vi "Main.vi"() -> ()   [LabVIEW 2024]
uses:
  <vilib>/NI/Modbus Library/API/Master/Modbus Master.lvclass
  Adams Library/6017/Support VIs/Range.ctl
  Adams Library/6224/Support VIs/AO Voltage Range.ctl
  <vilib>/addons/_JKI Toolkits/State Machine/_JKI_lib_State_Machine.llb/Select State(s)_err__jki_lib_state_machine.vi
  <vilib>/numeric/Random Number (Range) DBL.vi
  <vilib>/Utility/file.llb/Write Delimited Spreadsheet (DBL).vi
  <vilib>/Utility/file.llb/Write Delimited Spreadsheet (string).vi
  <userlib>/_OpenG.lib/appcontrol/appcontrol.llb/openg_application_control.lvlib
panel:
  out "Temperature":dbl format="%#_g °C"
  out "ICM Test":dbl(slide)=1.0 scale=0.0..100.0
  in  "Log File Name":string
  in  "Log Data":bool
  in  "Load Enable":bool
  out ">14µ":dbl
  out ">6µ":dbl
  out ">4µ":dbl
  out "Flow Rate":dbl[unit] format="%#_gl/m"
  in  "Load Percentage":u32(slide)=1 scale=0.0..100.0
  out "Post Cooler Temp":dbl format="%#.2g °C"
  out "Load Manifold Temp":dbl format="%#.2g °C"
  out "Motor Temp":dbl format="%#.2g °C"
  out "Load Pressure":dbl format="%#.2g bar"
  out "Cardev Pressure":dbl format="%#.2g bar"
  out "Post Filter Pressure":dbl format="%#.2g bar"
  out "Prefilter Pressure":dbl format="%#.2g bar"
  out "Temperatures":T1(graph) caption="Waveform Chart - Dark"
  in  "Close Button":bool
  out "Pressures":T2(graph) caption="Waveform Chart - Dark"
  # "HPU VALIDATION TEST"
  # "Temperatures"
  # "Pressures"
  # "Load Control"
  # "Flow Meter"
  # "ICM"
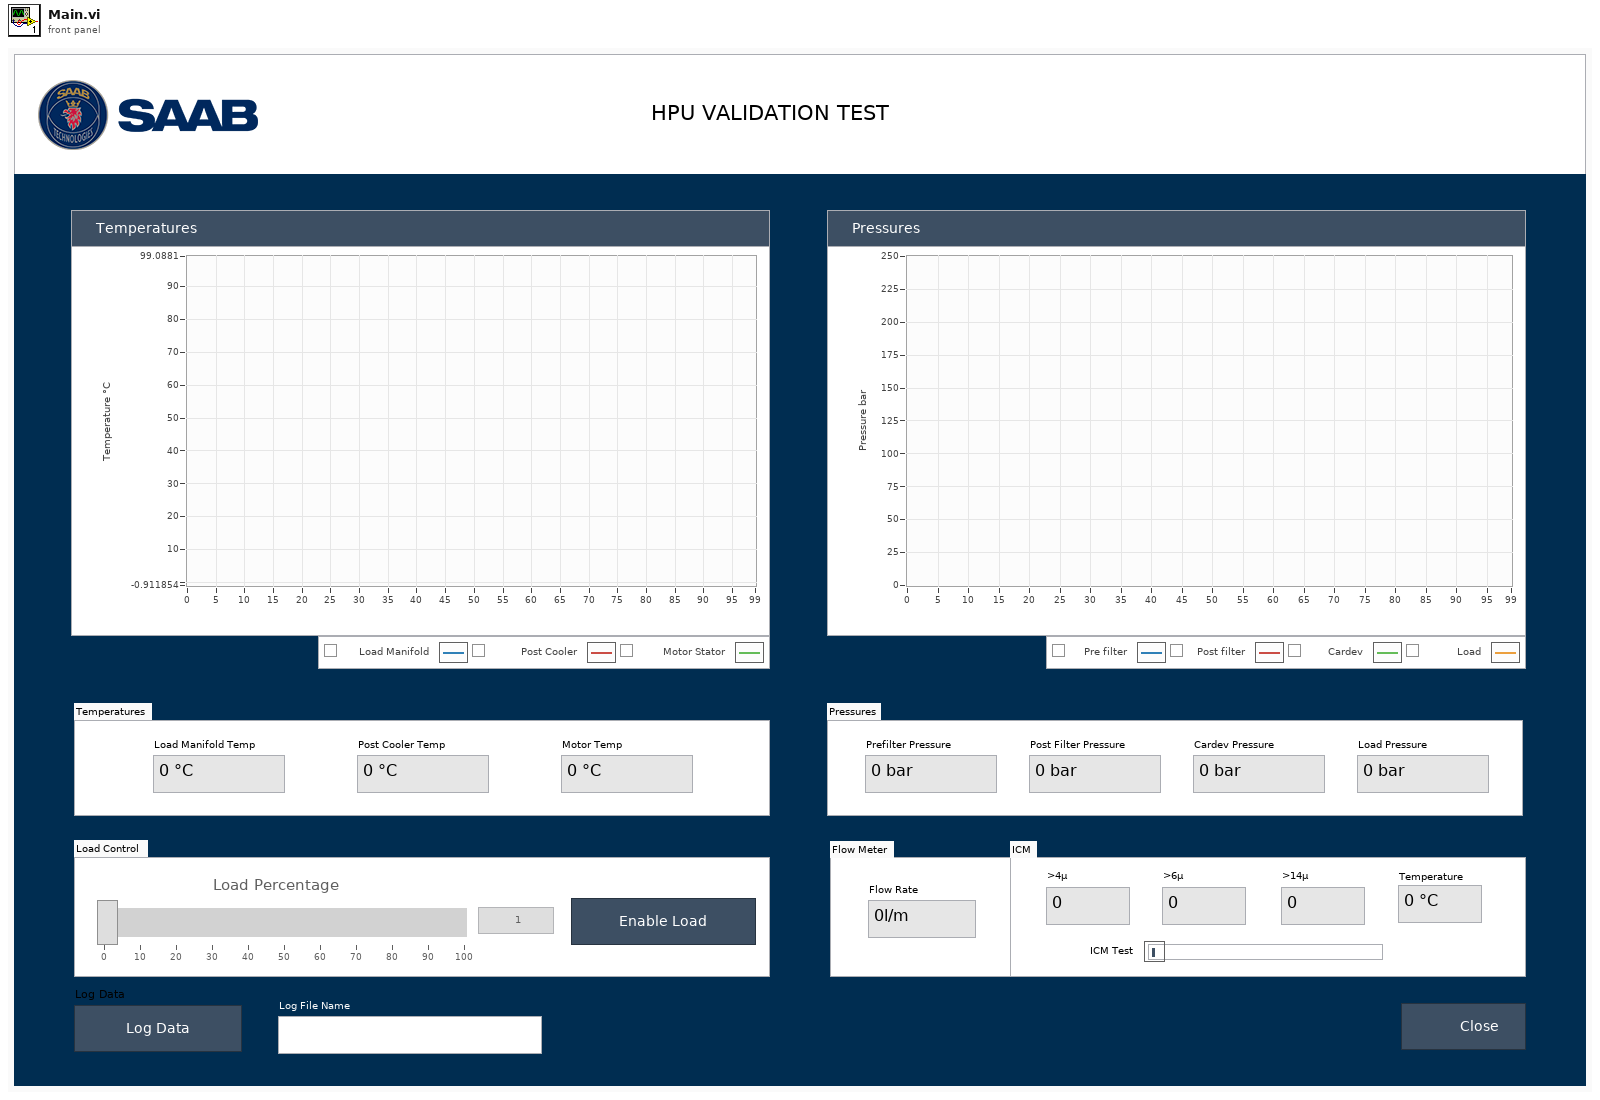
[diagram p1: front panel]
types:
  T1 = cluster{"Numeric":dbl, "Numeric":dbl, "Temperature °C":dbl}
  T2 = cluster{"Pressure bar":dbl, "Pressure bar":dbl, "Pressure bar":dbl, "Pressure bar":dbl}
  T3 = enum32{"Invalid", "Standard", "Closed", "Hidden", "Minimized", "Maximized"}
  T4 = enum32{"invalid app kind", "Development System", "Run Time System", "Student Edition", "Embedded LabVIEW", "Evaluation", "Custom"}
  T5 = cluster{"Numeric":dbl, "Numeric":dbl, "Temperature °C":dbl}[]
  T6 = cluster{"Pressure bar":dbl, "Pressure bar":dbl, "Pressure bar":dbl, "Pressure bar":dbl}[]
  T7 = enum8{"Enabled", "Disabled", "Disabled and Grayed Out"}
  T8 = typedef "Range.ctl" = u16
  T9 = cluster{"Core":cluster{"Current VI Reference":refnum<vi>, "Close Panel on Exit?":bool}, "6017 Ref":refnum<class "Modbus Master.lvclass">, "6224 Ref":refnum<class "Modbus Master.lvclass">, "AI Measurment":dbl[], "Channel Ranges":T8[], "Timestamp":dbl, "Simulate Data":bool, "Results File Path":path, "Log Data":dbl[], "Write Data":bool, "Load Percentage":u32, "ICM Ref":refnum<class "Modbus Master.lvclass">}
  T10 = cluster{"Current VI Reference":refnum<vi>, "Close Panel on Exit?":bool}
  T11 = typedef "AO Voltage Range.ctl" = u16
  T12 = cluster{"Temperature °C":dbl, "Temperature °C":dbl, "Temperature °C":dbl}
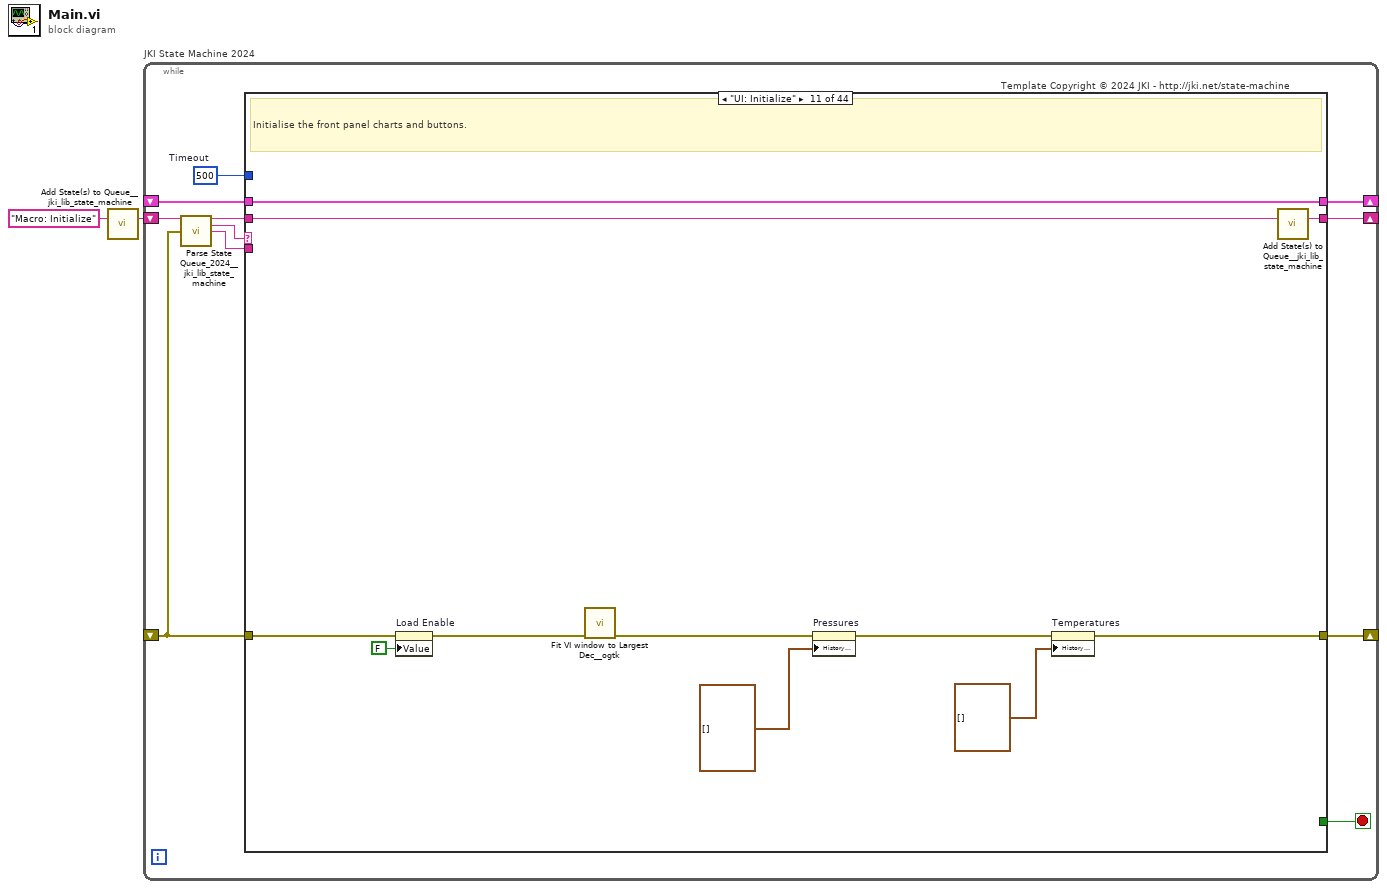
[diagram p0: block diagram]
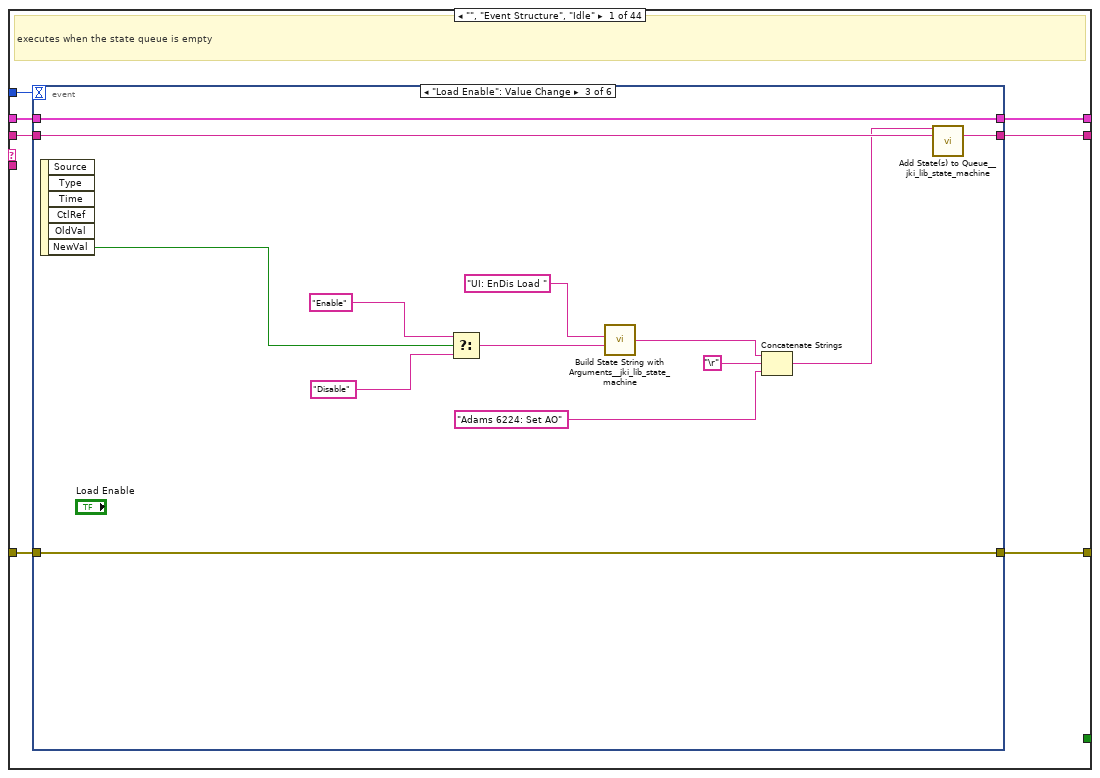
[diagram p2: hidden frame]
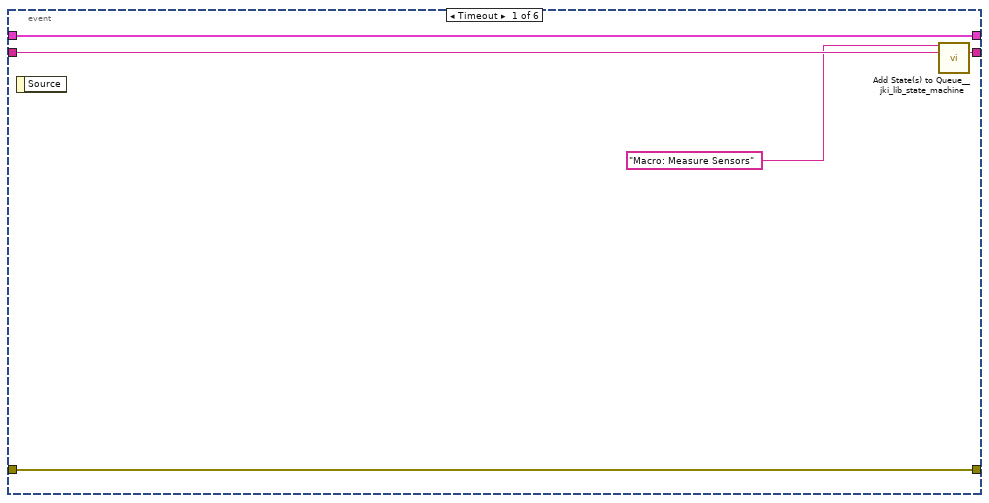
[diagram p3: hidden frame]
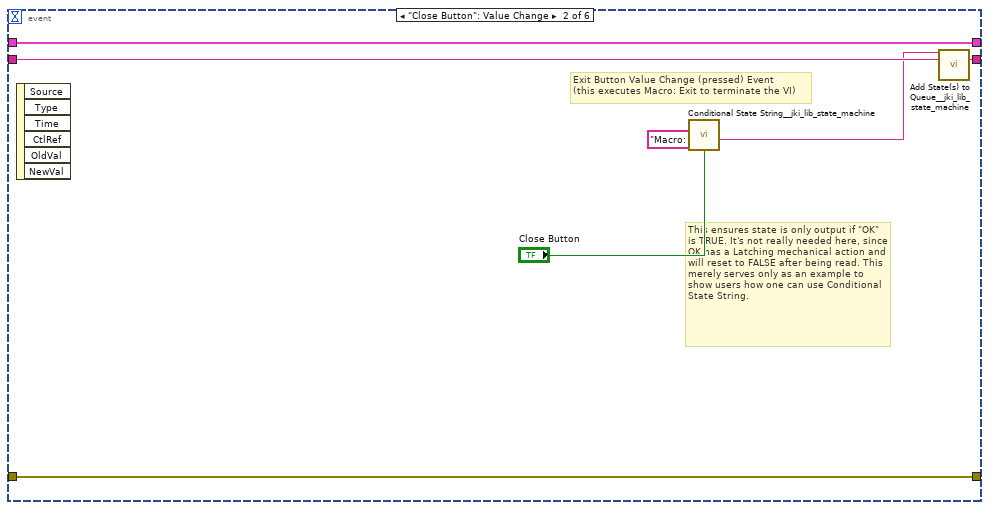
[diagram p4: hidden frame]
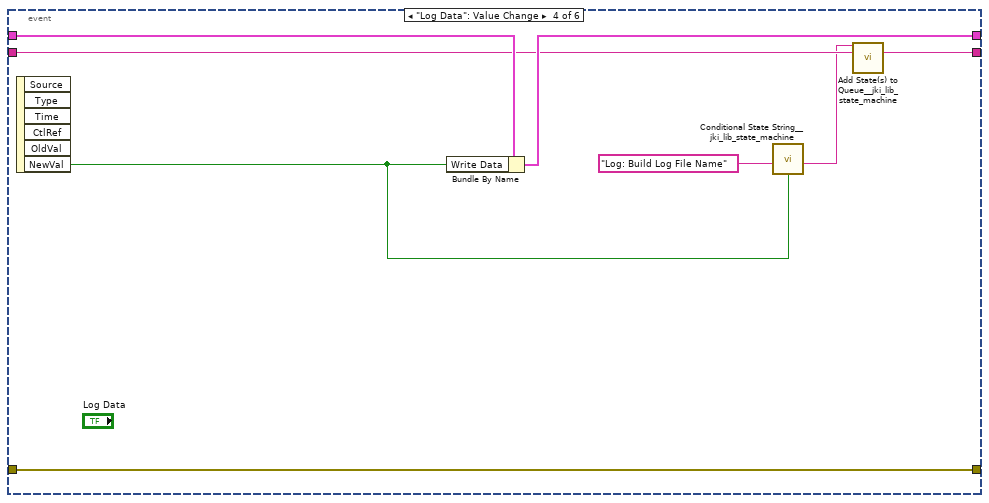
[diagram p5: hidden frame]
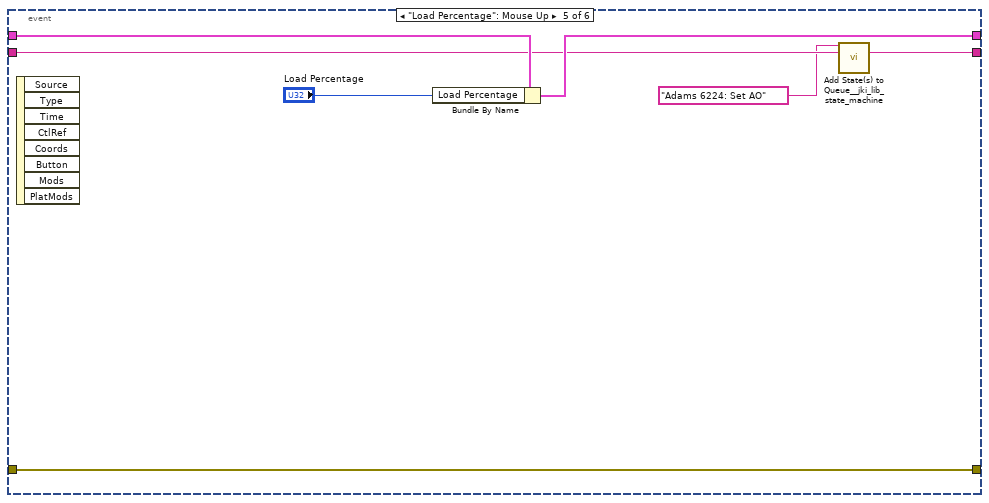
[diagram p6: hidden frame]
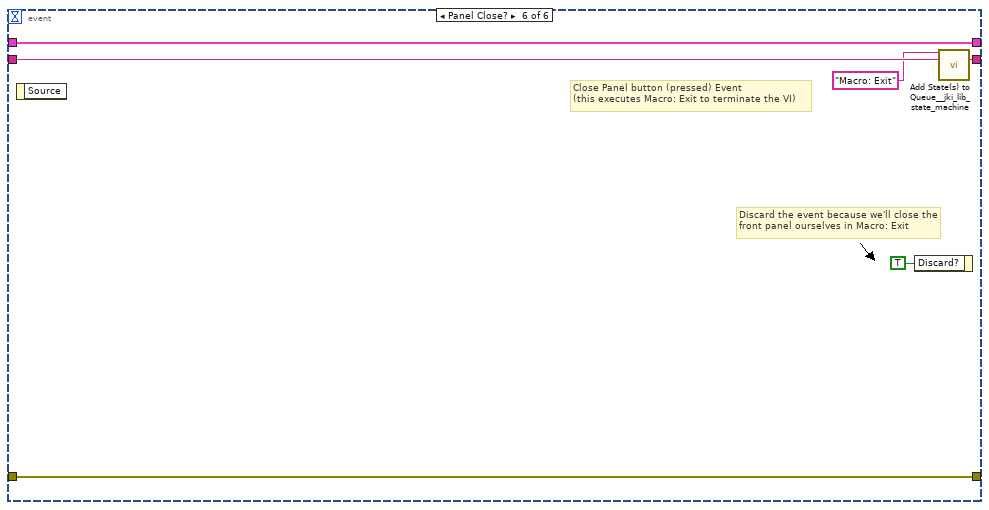
[diagram p7: hidden frame]
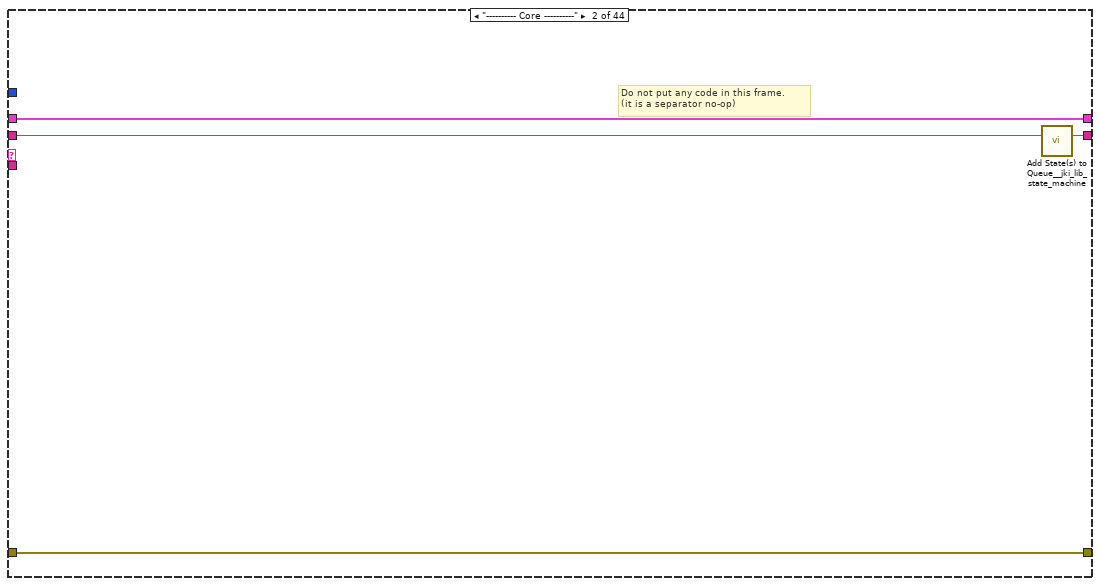
[diagram p8: hidden frame]
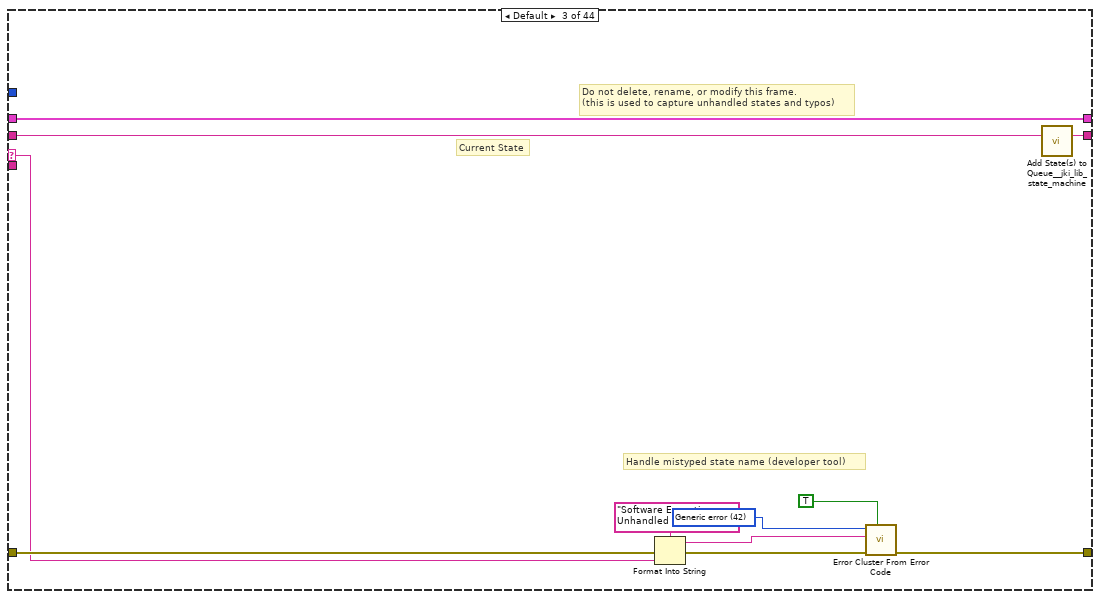
[diagram p9: hidden frame]
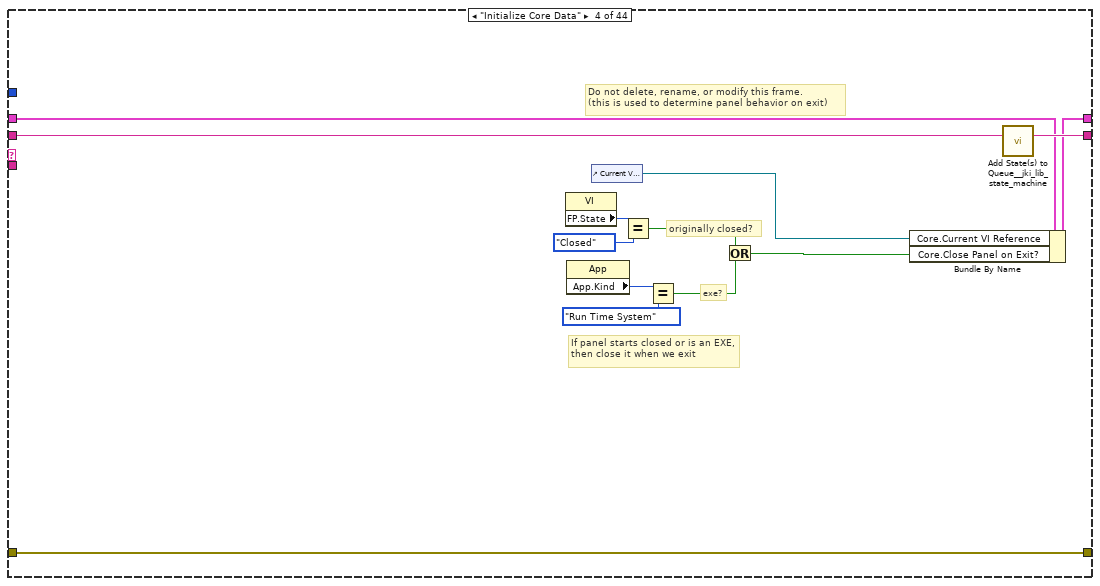
[diagram p10: hidden frame]
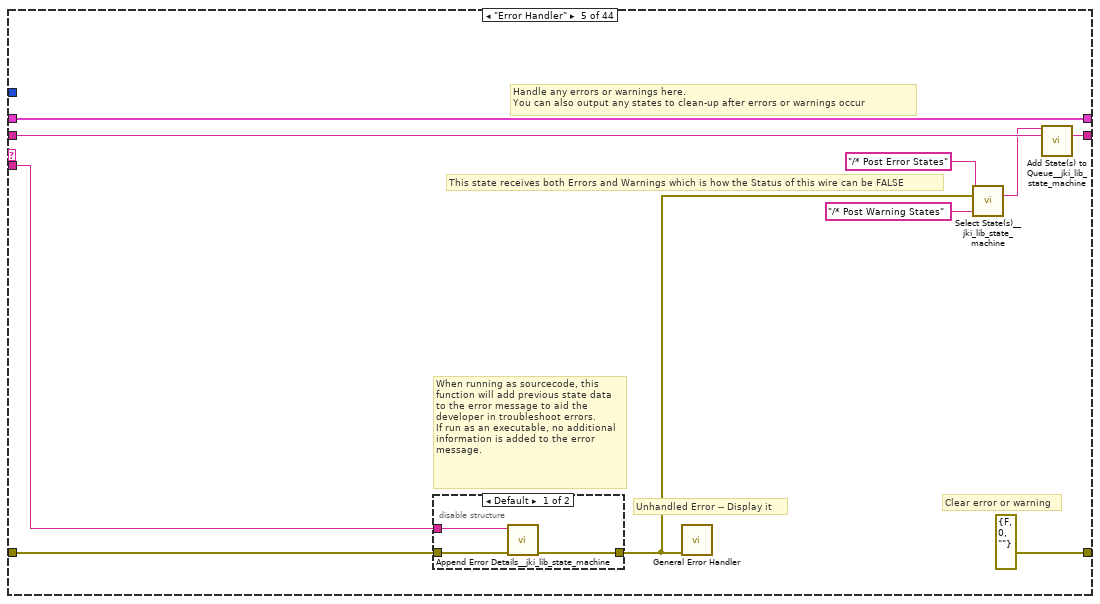
[diagram p11: hidden frame]
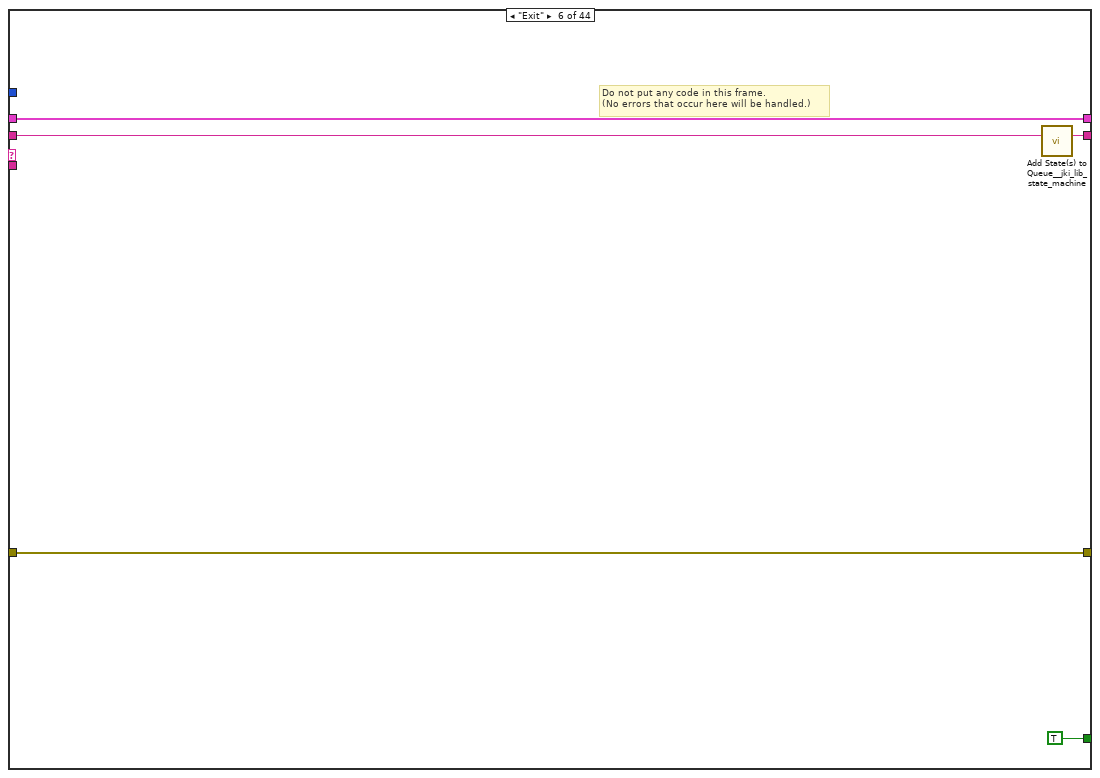
[diagram p13: hidden frame]
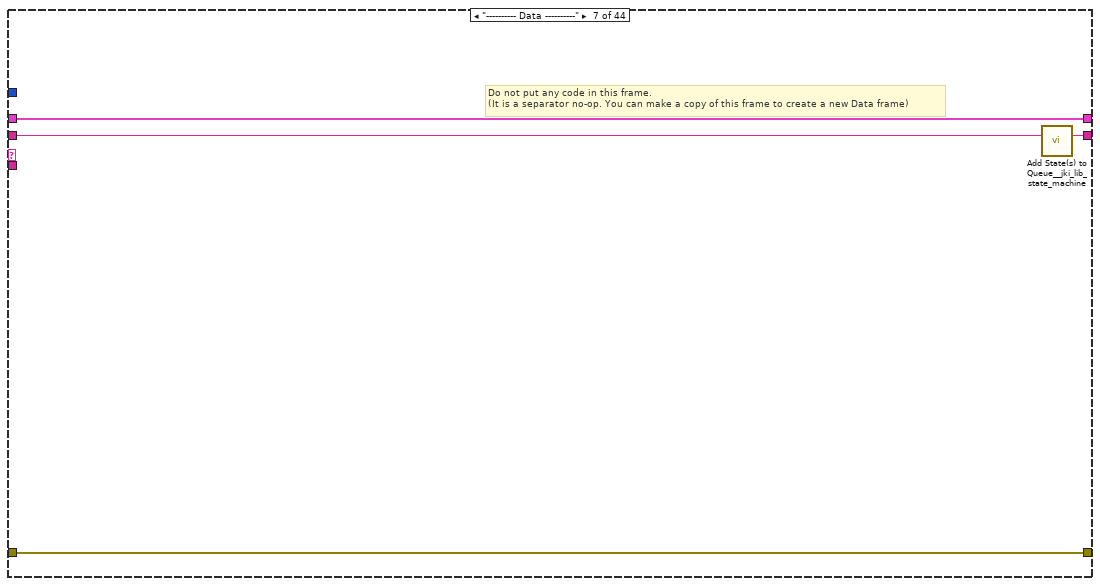
[diagram p14: hidden frame]
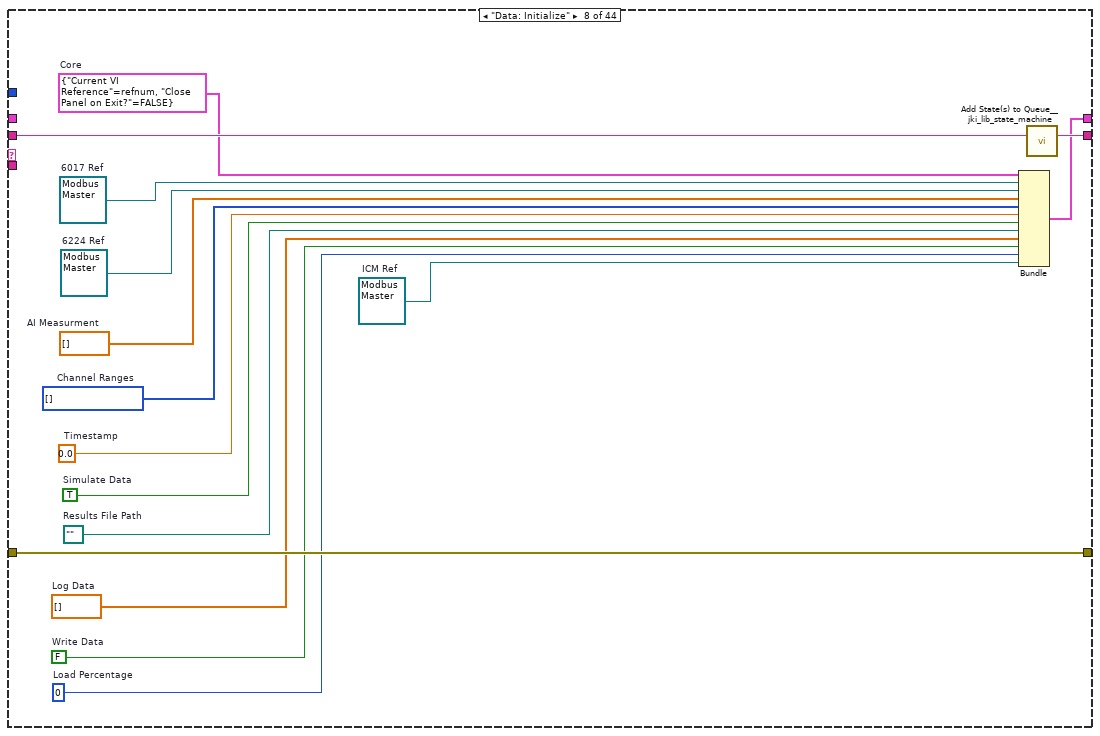
[diagram p15: hidden frame]
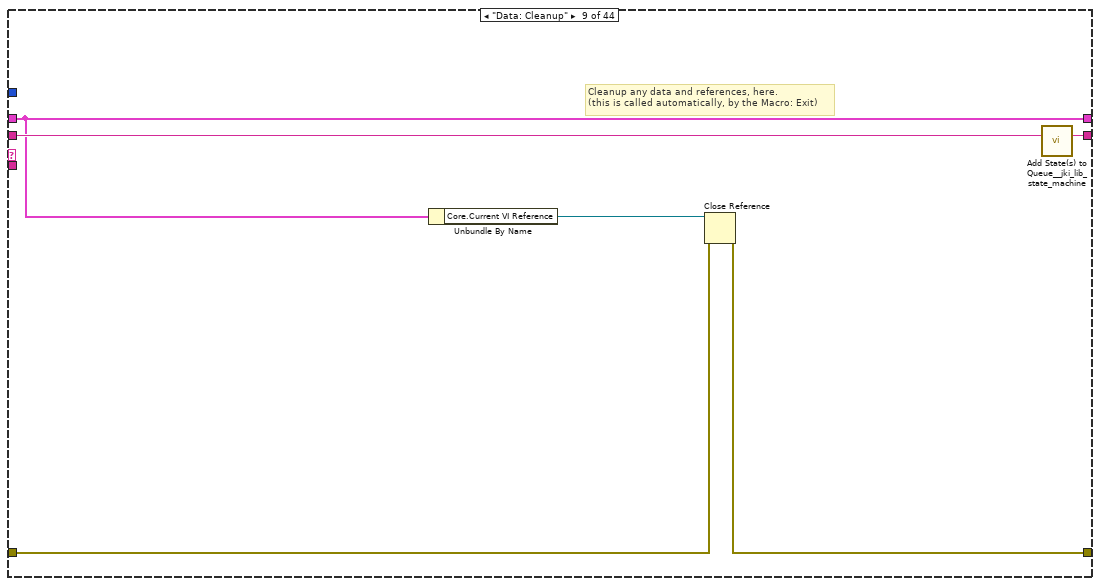
[diagram p16: hidden frame]
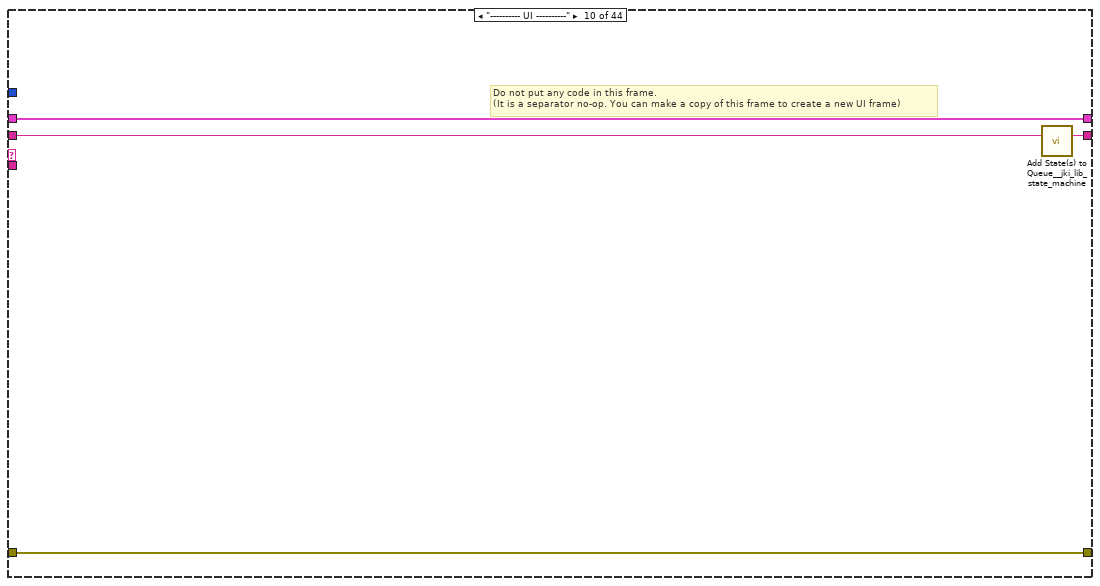
[diagram p17: hidden frame]
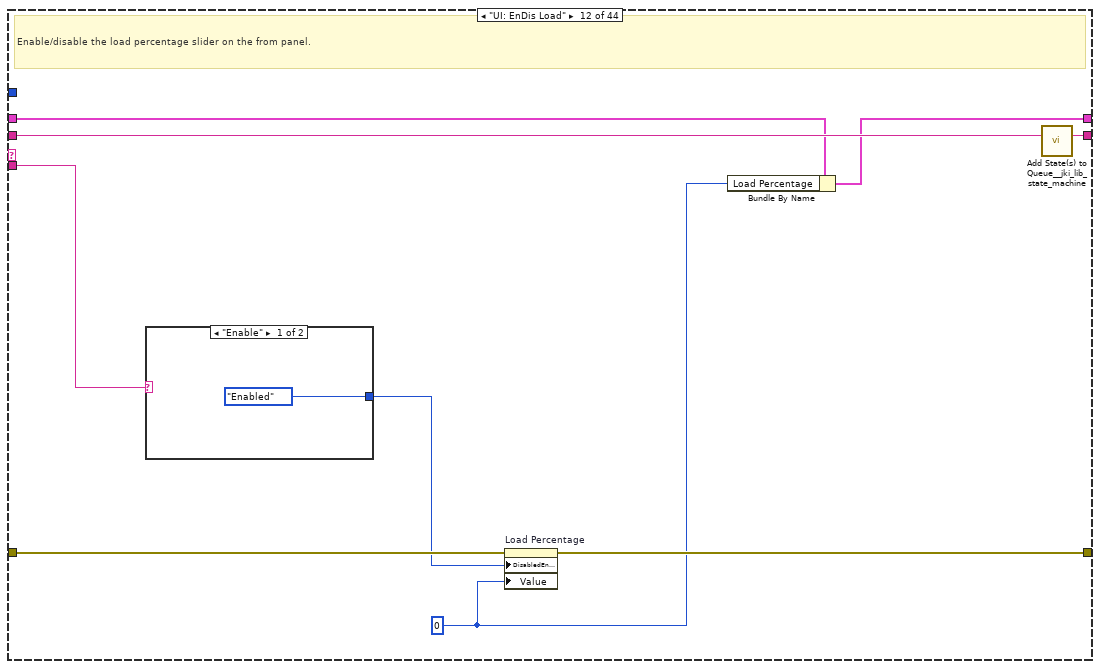
[diagram p18: hidden frame]
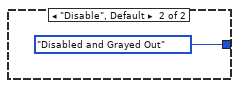
[diagram p19: hidden frame]
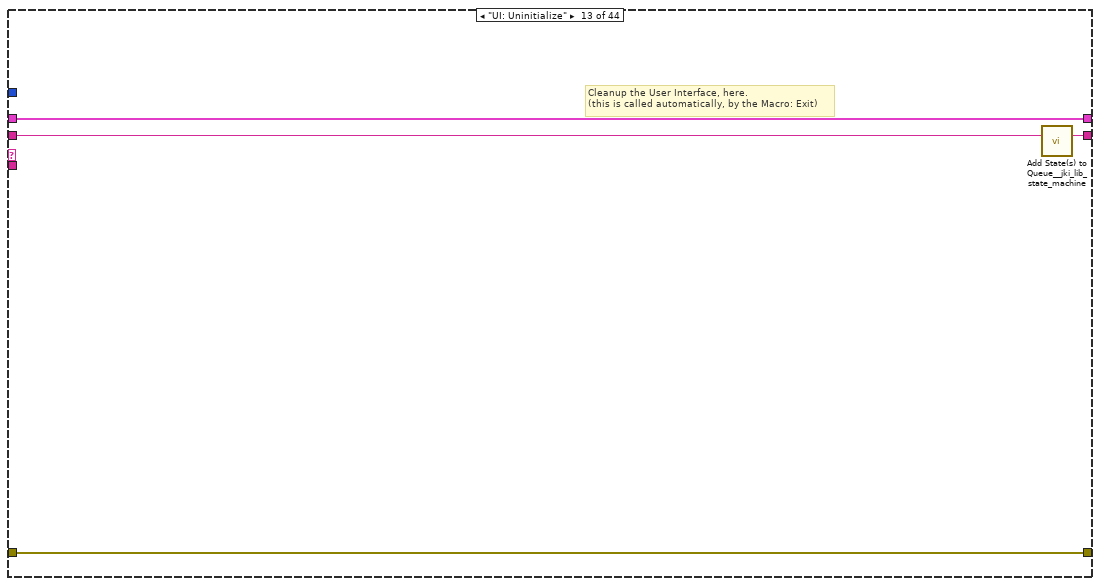
[diagram p20: hidden frame]
diagram:
  n1 = call <vilib>:"Add State(s) to Queue__jki_lib_state_machine.vi"("State(s) in (\"\")"="Macro: Initialize") -> ("States Out"=w2:string)  [unwired: 14 in]
  n2 = while "JKI State Machine 2024" {
    shift-right: [w6] -> _
    shift-left: _ -> [w5]
    shift-right: [w9] -> _
    shift-left: _ -> [w3]
    shift-right: [w8] -> _
    shift-left: w2 -> [w10]
    stop <- w7 stop-if-true
    w4 = 500  # Timeout
    # "Template Copyright © 2024 JKI - http://jki.net/state-machine"
    n3 = call <vilib>:"Parse State Queue_2024__jki_lib_state_machine.vi"("State Queue"=w10, "Error In (no error)"=w3) -> ("Remaining States"=w12:string, "Current State"=w13:string, "Arguments"=w11:string)  [unwired: 11 in]
    n4 = case shown="\"UI: Initialize\"" w13 {
      selector: w13 -> [_ _ w71 _ _ _ _ _ _ _ _ _ _ _ _ _ _ _ _ _ _ _ _ _ _ _ _ _ _ _ _ _ _ _ _ _ _ _ _ _ _ _ _ _]
      tunnel: w12 -> [w20 w70 w75 w94 w104 w113 w117 w133 w139 w143 w154 w163 w169 w175 w186 w255 w260 w265 w274 w278 w286 w299 w373 w384 w396 w400 w408 w424 w432 w436 w455 w459 w476 w480 w488 w496 w509 w518 w527 w531 w541 w564 w568 w572]
      tunnel: w11 -> [_ _ _ _ w99 _ _ _ _ _ _ w158 _ w170 w180 _ _ _ _ _ _ _ _ w376 _ _ _ _ _ _ _ _ _ _ _ _ _ _ _ _ _ _ _ _]
      tunnel: w5 -> [w18 w67 w73 w87 w101 w111 w114 _ w134 w140 w152 w157 w167 w173 w182 w252 w257 w262 w272 w275 w281 w295 w368 w379 w391 w397 w403 w421 w426 w433 w441 w456 w462 w477 w483 w493 w506 w515 w524 w528 w535 w555 w565 w569]
      tunnel: [w17 w68 w77 w91 errorcluster {"status"=FALSE, "code"=0, "source"=""} ("error out") w110 w115 w130 w135 w141 w145 w160 w166 w171 w183 w253 w258 w263 w269 w276 w283 w292 w369 w382 w393 w398 w404 w420 w429 w434 w453 w457 w474 w478 w484 w492 w505 w514 w523 w529 w536 w551 w566 w570] -> w9
      tunnel: w3 -> [w14 w68 w76 w91 w100 w110 w115 w130 w136 w141 w150 w161 w166 w172 w184 w253 w258 w263 w269 w276 w284 w297 w371 w380 w394 w398 w405 w419 w430 w434 w453 w457 w474 w478 w486 w491 w504 w513 w522 w529 w539 w552 w566 w570]
      tunnel: [w19 w69 w74 w93 w103 w112 w116 w132 w138 w142 w153 w162 w168 w174 w185 w254 w259 w264 w273 w277 w285 w298 w372 w383 w395 w399 w407 w423 w431 w435 w454 w458 w475 w479 w487 w495 w508 w517 w526 w530 w540 w563 w567 w571] -> w8
      tunnel: [_ _ _ _ _ TRUE _ _ _ _ _ _ _ _ _ _ _ _ _ _ _ _ _ _ _ _ _ _ _ _ _ _ _ _ _ _ _ _ _ _ _ _ _ _] -> w7
      tunnel: [w16 w67 w73 w92 w101 w111 w114 w131 w134 w140 w152 w156 w167 w173 w182 w252 w257 w262 w272 w275 w280 w294 w367 w377 w390 w397 w402 w422 w425 w433 w440 w456 w461 w477 w482 w494 w507 w516 w525 w528 w534 w554 w565 w569] -> w6
      tunnel: w4 -> [w15 _ _ _ _ _ _ _ _ _ _ _ _ _ _ _ _ _ _ _ _ _ _ _ _ _ _ _ _ _ _ _ _ _ _ _ _ _ _ _ _ _ _ _]
      frame "", "Event Structure", "Idle" {
        # "executes when the state queue is empty"
        n5 = event shown="[2] \"Load Enable\": Value Change" {
          selector: _ -> [_ _ _ _ _ _]
          dyn-events: _ -> [_ _ _ _ _ _]
          timeout: w15 -> [_ _ _ _ _ _]
          tunnel: w20 -> [w25 w32 w43 w49 w55 w66]
          tunnel: [w24 w31 w44 w50 w56 w65] -> w19
          tunnel: w18 -> [w22 w29 w35 w52 w58 w63]
          tunnel: [w23 w30 w45 w53 w60 w64] -> w17
          tunnel: w14 -> [w23 w30 w45 w53 w60 w64]
          tunnel: [w22 w29 w35 w51 w59 w63] -> w16
          event Timeout {
            n6 = event-data() -> ()  [unwired: 1 in, 1 out]
            n7 = call <vilib>:"Add State(s) to Queue__jki_lib_state_machine.vi"("State(s) in Front (\"\")"="Macro: Measure Sensors", "State(s) in (\"\")"=w25) -> ("States Out"=w24:string)  [unwired: 13 in]
          }
          event "Close Button": Value Change {
            # "This ensures state is only output if \"OK\" is TRUE. It's not really needed here, since OK has a Latching mechanical action and will reset to FALSE after being read. This merely serves only as an example to show users how one can use Conditional State String."
            # "Exit Button Value Change (pressed) Event\n(this executes Macro: Exit to terminate the VI)"
            n8 = event-data() -> ()  [unwired: 1 in, 6 out]
            n9 = call <vilib>:"Conditional State String__jki_lib_state_machine.vi"("Do State(s)?"="Close Button", "State"="Macro: Exit") -> ("State Out"=w27:string)  [unwired: 7 in]
            n10 = call <vilib>:"Add State(s) to Queue__jki_lib_state_machine.vi"("State(s) in Front (\"\")"=w27, "State(s) in (\"\")"=w32) -> ("States Out"=w31:string)  [unwired: 13 in]
          }
          event "Load Enable": Value Change {
            n11 = event-data() -> ("NewVal"=w42:bool)  [unwired: 1 in, 5 out]
            n12 = Select(t="Enable", s=w42, f="Disable") -> (s? t:f=w40:string)
            n13 = call <vilib>:"Build State String with Arguments__jki_lib_state_machine.vi"("Arguments (\"\")"=w40, "State"="UI: EnDis Load ") -> ("State with Arguments"=w34:string)  [unwired: 4 in]
            n14 = Concatenate Strings(w34, "\r", "Adams 6224: Set AO") -> (w37:string)
            n15 = call <vilib>:"Add State(s) to Queue__jki_lib_state_machine.vi"("State(s) in Front (\"\")"=w37, "State(s) in (\"\")"=w43) -> ("States Out"=w44:string)  [unwired: 13 in]
          }
          event "Log Data": Value Change {
            n16 = event-data() -> ("NewVal"=w48:bool)  [unwired: 1 in, 5 out]
            n17 = Bundle By Name(cluster=w52, "Write Data"=w48) -> (w51:T9)
            n18 = call <vilib>:"Conditional State String__jki_lib_state_machine.vi"("Do State(s)?"=w48, "State"="Log: Build Log File Name") -> ("State Out"=w46:string)  [unwired: 7 in]
            n19 = call <vilib>:"Add State(s) to Queue__jki_lib_state_machine.vi"("State(s) in Front (\"\")"=w46, "State(s) in (\"\")"=w49) -> ("States Out"=w50:string)  [unwired: 13 in]
          }
          event "Load Percentage": Mouse Up {
            n20 = event-data() -> ()  [unwired: 1 in, 8 out]
            n21 = Bundle By Name(cluster=w58, "Load Percentage"="Load Percentage") -> (w59:T9)
            n22 = call <vilib>:"Add State(s) to Queue__jki_lib_state_machine.vi"("State(s) in Front (\"\")"="Adams 6224: Set AO", "State(s) in (\"\")"=w55) -> ("States Out"=w56:string)  [unwired: 13 in]
          }
          event Panel Close? {
            # "Discard the event because we'll close the front panel ourselves in Macro: Exit"
            # "Close Panel button (pressed) Event\n(this executes Macro: Exit to terminate the VI)"
            n23 = event-data() -> ()  [unwired: 1 in, 1 out]
            n24 = event-data("Discard?"=TRUE) -> ()  [unwired: 1 in, 1 out]
            n25 = call <vilib>:"Add State(s) to Queue__jki_lib_state_machine.vi"("State(s) in Front (\"\")"="Macro: Exit", "State(s) in (\"\")"=w66) -> ("States Out"=w65:string)  [unwired: 13 in]
          }
        }
      }
      frame "---------- Core ----------" {
        # "Do not put any code in this frame.\n(it is a separator no-op)"
        n26 = call <vilib>:"Add State(s) to Queue__jki_lib_state_machine.vi"("State(s) in (\"\")"=w70) -> ("States Out"=w69:string)  [unwired: 14 in]
      }
      frame Default {
        w80 = 42 items=["No error", "Argument error", "Memory is full", "Out of zone", "End of file", "File already open", "Generic file I/O error", "File not found", "File permission error", "Disk is full", "Duplicate path", "Too many files open", "System feature not enabled", "Resource file not found", "Cannot add resource", "Resource not found", "Image not found", "Image memory error", "Pen does not exist", "Config type invalid", "Config token not found", "Config parse error", "Config memory error", "Bad external code format", "Bad external code offset", "External code not present", "Null window", "Destroy window error", "Null menu", "Print aborted", "Bad print record", "Print driver error", "Windows error during printing", "Memory error during printing", "Print dialog error", "Generic print error", "Invalid device refnum", "Device not found", "Device parameter error", "Device unit error", "Cannot open device", "Device call aborted", "Generic error", "Cancelled by user", "Object ID too low", "Object ID too high", "Object not in heap", "Unknown heap", "Unknown object (invalid DefProc)", "Unknown object (DefProc not in table)", "Message out of range", "Invalid (null) method", "Unknown message", "Manager call not supported", "Bad address", "Network operation in progress", "Network operation timed out", "Connection is busy", "Network attribute not supported", "Network error", "Address in use", "System out of memory", "Connection aborted", "Connection refused", "Not connected", "Already connected", "Connection closed", "Initialization error (interapplication manager)", "Bad occurrence", "Wait on unbound occurrence handler", "Occurrence queue overflow", "Datalog type conflict", "Unused", "Unrecognized type (interapplication manager)", "Memory corrupt", "Failed to make temporary DLL", "Old CIN version", "Drag socket not found", "Failed to load drop-object", "Failed to register OLE object", "Failed to release OLE object", "Format specifier type mismatch", "Unknown format specifier", "Too few format specifiers", "Too many format specifiers", "Scan failed", "Newer CIN version", "Error converting to variant", "Runtime menu error", "Password tampered", "Variant attribute not found", "Incompatible variant data type", "Event data is not available", "Event Store is not present", "Occurrence is not found", "Event Queue is not created", "Event info is not available", "Refnum passed is NULL", "Error retrieving Class GUID", "Error retrieving CoClass GUID", "Error retrieving TypeLib GUID.", "Bad built application magic bytes.", "Specific driver is different from the specific driver associated with the Logical Name.", "There is no session opened to the class driver.", "Max Error", "MAX - Error with config objects", "MAX - Error loading configuration", "MAX - Group not supported"]
        # "Current State"
        # "Do not delete, rename, or modify this frame.\n(this is used to capture unhandled states and typos)"
        # "Handle mistyped state name (developer tool)"
        n27 = Format Into String(format string="Software Exception: Unhandled State \"%s\"." ("message"), error in=w76, w71) -> (resulting string=w79:string, error out=w78:errorcluster)  [unwired: 1 in]
        n28 = call <vilib>:"Error Cluster From Error Code.vi"("show call chain? (False)"=TRUE, "error in (no error)"=w78, "error message (\"\")"=w79, "error code (0)"=w80) -> ("error out"=w77:errorcluster)  [unwired: 5 in]
        n29 = call <vilib>:"Add State(s) to Queue__jki_lib_state_machine.vi"("State(s) in (\"\")"=w75) -> ("States Out"=w74:string)  [unwired: 14 in]
      }
      frame "Initialize Core Data" {
        # "Do not delete, rename, or modify this frame.\n(this is used to determine panel behavior on exit)"
        # "originally closed?"
        # "exe?"
        # "If panel starts closed or is an EXE, then close it when we exit"
        n30 = property class="VI"() -> ("FP.State"=w84:T3)  [unwired: 2 in, 2 out]
        n31 = property class="App"() -> ("App.Kind"=w90:T4)  [unwired: 2 in, 2 out]
        n32 = control-ref of="Current VI Reference"() -> (w85:refnum<vi>)
        n33 = Equal?(x=w84, y=T3."Closed" ("Front Panel Window:State")) -> (x = y?=w82:bool)
        n34 = Equal?(x=w90, y=T4."Run Time System" ("Application:Kind")) -> (x = y?=w88:bool)
        n35 = Or(x=w82, y=w88) -> (x .or. y?=w86:bool)
        n36 = Bundle By Name(cluster=w87, "Core.Current VI Reference"=w85, "Core.Close Panel on Exit?"=w86) -> (w92:T9)
        n37 = call <vilib>:"Add State(s) to Queue__jki_lib_state_machine.vi"("State(s) in (\"\")"=w94) -> ("States Out"=w93:string)  [unwired: 14 in]
      }
      frame "Error Handler" {
        # "When running as sourcecode, this function will add previous state data to the error message to aid the developer in troubleshoot errors.\nIf run as an executable, no additional information is added to the error message."
        # "This state receives both Errors and Warnings which is how the Status of this wire can be FALSE"
        # "Unhandled Error -- Display it"
        # "Handle any errors or warnings here.\nYou can also output any states to clean-up after errors or warnings occur"
        # "Clear error or warning"
        n38 = disable-structure shown="Default" {
          disable-tunnel: w100 -> [w107 w108]
          disable-tunnel: w99 -> [w106 _]
          disable-tunnel: [w105 w108] -> w98
          frame condition #0 (active) {
            n39 = call <vilib>:"Append Error Details__jki_lib_state_machine.vi"("error in (no error)"=w107, "Previous State and Argument(s)"=w106) -> ("error out"=w105:errorcluster)  [unwired: 9 in]
          }
          frame condition #1 {
          }
        }
        n40 = call <vilib>:"General Error Handler.vi"("error in (no error)"=w98) -> ()  [unwired: 10 in, 5 out]
        n41 = call-poly <vilib>:"Select State(s)__jki_lib_state_machine.vi"("State(s) if True (\"\")"="/* Post Error States", "Select"=w98, "State(s) if False (\"\")"="/* Post Warning States") -> ("States Out"=w96:string)  [unwired: 12 in]
        n42 = call <vilib>:"Add State(s) to Queue__jki_lib_state_machine.vi"("State(s) in Front (\"\")"=w96, "State(s) in (\"\")"=w104) -> ("States Out"=w103:string)  [unwired: 13 in]
      }
      frame "Exit" {
        # "Do not put any code in this frame.\n(No errors that occur here will be handled.)"
        n43 = call <vilib>:"Add State(s) to Queue__jki_lib_state_machine.vi"("State(s) in (\"\")"=w113) -> ("States Out"=w112:string)  [unwired: 14 in]
      }
      frame "---------- Data ----------" {
        # "Do not put any code in this frame.\n(It is a separator no-op. You can make a copy of this frame to create a new Data frame)"
        n44 = call <vilib>:"Add State(s) to Queue__jki_lib_state_machine.vi"("State(s) in (\"\")"=w117) -> ("States Out"=w116:string)  [unwired: 14 in]
      }
      frame "Data: Initialize" {
        w118 = refnum<class "Modbus Master.lvclass"> refnum  # ICM Ref
        w119 = u32 0  # Load Percentage
        w120 = FALSE  # Write Data
        w121 = dbl[] []  # Log Data
        w122 = path ""  # Results File Path
        w123 = TRUE  # Simulate Data
        w124 = 0.0  # Timestamp
        w125 = T8[] [] items=["+-150mV"=259, "+-500mV"=260, "0~150mV"=261, "0~500mV"=262, "+-1V"=320, "+-5V"=322, "+-10V"=323, "0~1V"=325, "0~5V"=327, "0~10V"=328, "+-20mA"=385, "4~20mA"=384, "0~20mA"=386]  # Channel Ranges
        w126 = dbl[] []  # AI Measurment
        w127 = refnum<class "Modbus Master.lvclass"> refnum  # 6224 Ref
        w128 = refnum<class "Modbus Master.lvclass"> refnum  # 6017 Ref
        w129 = T10 {"Current VI Reference"=refnum, "Close Panel on Exit?"=FALSE}  # Core
        n45 = Bundle("Core"=w129, "6017 Ref"=w128, "6224 Ref"=w127, "AI Measurment"=w126, "Channel Ranges"=w125, "Timestamp"=w124, "Simulate Data"=w123, "Results File Path"=w122, "Log Data"=w121, "Write Data"=w120, "Load Percentage"=w119, "ICM Ref"=w118) -> (w131:T9)  [unwired: 1 in]
        n46 = call <vilib>:"Add State(s) to Queue__jki_lib_state_machine.vi"("State(s) in (\"\")"=w133) -> ("States Out"=w132:string)  [unwired: 14 in]
      }
      frame "Data: Cleanup" {
        # "Cleanup any data and references, here.\n(this is called automatically, by the Macro: Exit)"
        n47 = Unbundle By Name(w134) -> ("Core.Current VI Reference"=w137:refnum<vi>)
        n48 = Close Reference(reference=w137, error in (no error)=w136) -> (error out=w135:errorcluster)
        n49 = call <vilib>:"Add State(s) to Queue__jki_lib_state_machine.vi"("State(s) in (\"\")"=w139) -> ("States Out"=w138:string)  [unwired: 14 in]
      }
      frame "---------- UI ----------" {
        # "Do not put any code in this frame.\n(It is a separator no-op. You can make a copy of this frame to create a new UI frame)"
        n50 = call <vilib>:"Add State(s) to Queue__jki_lib_state_machine.vi"("State(s) in (\"\")"=w143) -> ("States Out"=w142:string)  [unwired: 14 in]
      }
      frame "UI: Initialize" {
        # "Initialise the front panel charts and buttons."
        n51 = property on="Load Enable" class="Bool (strict)"(error in=w150, "Value"=FALSE ("Load Enable")) -> (error out=w151:errorcluster)  [unwired: 1 in, 1 out]
        n52 = call <userlib>:"Fit VI window to Largest Dec__ogtk.vi"("error in (no error)"=w151) -> ("error out"=w148:errorcluster)  [unwired: 5 in, 1 out]
        n53 = property on="Pressures" class="WFChart (strict)"(error in=w148, "History Data"=T6 []) -> (error out=w146:errorcluster)  [unwired: 1 in, 1 out]
        n54 = property on="Temperatures" class="WFChart (strict)"(error in=w146, "History Data"=T5 []) -> (error out=w145:errorcluster)  [unwired: 1 in, 1 out]
        n55 = call <vilib>:"Add State(s) to Queue__jki_lib_state_machine.vi"("State(s) in (\"\")"=w154) -> ("States Out"=w153:string)  [unwired: 14 in]
      }
      frame "UI: EnDis Load" {
        w155 = u32 0 ("Load Percentage")
        # "Enable/disable the load percentage slider on the from panel."
        n56 = case shown="\"Enable\"" w158 {
          tunnel: [T7."Enabled" ("Disabled") T7."Disabled and Grayed Out" ("Disabled")] -> w159
          frame "Enable" {
          }
          frame "Disable", Default {
          }
        }
        n57 = property on="Load Percentage" class="Slide (strict)"(error in=w161, "DisabledEnum"=w159, "Value"=w155) -> (error out=w160:errorcluster)  [unwired: 1 in, 1 out]
        n58 = Bundle By Name(cluster=w157, "Load Percentage"=w155) -> (w156:T9)
        n59 = call <vilib>:"Add State(s) to Queue__jki_lib_state_machine.vi"("State(s) in (\"\")"=w163) -> ("States Out"=w162:string)  [unwired: 14 in]
      }
      frame "UI: Uninitialize" {
        # "Cleanup the User Interface, here.\n(this is called automatically, by the Macro: Exit)"
        n60 = call <vilib>:"Add State(s) to Queue__jki_lib_state_machine.vi"("State(s) in (\"\")"=w169) -> ("States Out"=w168:string)  [unwired: 14 in]
      }
      frame "UI: Cursor Set" {
        # "Argument"
        # "Set and Unset Cursor Busy.\n(Usage: \"UI: Cursor Set >> Busy|Idle\")"
        n61 = case shown="\"Idle\", Default" w170 {
          tunnel: w172 -> [w177 w179]
          tunnel: [w176 w178] -> w171
          frame "Idle", Default {
            n62 = call <vilib>:"Unset Busy.vi"("error in (no error)"=w177) -> ("error out"=w176:errorcluster)  [unwired: 10 in]
          }
          frame "Busy" {
            n63 = call <vilib>:"Set Busy.vi"("error in (no error)"=w179) -> ("error out"=w178:errorcluster)  [unwired: 9 in, 1 out]
          }
        }
        n64 = call <vilib>:"Add State(s) to Queue__jki_lib_state_machine.vi"("State(s) in (\"\")"=w175) -> ("States Out"=w174:string)  [unwired: 14 in]
      }
      frame "UI: Front Panel State" {
        # "Argument"
        # "Set Front Panel Open or Closed\n(Usage: \"UI: Front Panel State >> Open|Close\")"
        n65 = Unbundle By Name(w182) -> ("Core.Current VI Reference"=w181:refnum<vi>)
        n66 = case shown="\"Minimize\", \"Minimized\"" w180 {
          tunnel: w184 -> [w192 w207 w218 w231 w244]
          tunnel: [w194 w208 w220 w233 w246] -> w183
          tunnel: w181 -> [w193 w205 w219 w232 w245]
          frame "Open", "Standard", Default {
            w187 = T3."Standard" ("State")
            n67 = property class="VI"(reference=w193, error in=w192) -> (reference out=w190:refnum<vi>, error out=w191:errorcluster, "FP.State"=w189:T3)
            n68 = Not Equal?(x=w189, y=w187) -> (x != y?=w188:bool)
            n69 = case shown="True" w188 {
              tunnel: [w198 w200] -> w194
              tunnel: w191 -> [w197 w200]
              tunnel: w190 -> [w196 _]
              tunnel: w187 -> [w195 _]
              frame True {
                n70 = invoke class="VI" method="FP.Open"(reference=w196, error in=w197, "Activate"=TRUE, "State"=w195) -> (error out=w198:errorcluster)  [unwired: 1 in, 4 out]
              }
              frame False {
              }
            }
          }
          frame "Close", "Closed" {
            n71 = property class="VI"(reference=w205, error in=w207) -> (reference out=w204:refnum<vi>, error out=w206:errorcluster, "FP.State"=w202:T3)
            n72 = Not Equal?(x=w202, y=T3."Closed" ("Front Panel Window:State")) -> (x != y?=w201:bool)
            n73 = case shown="True" w201 {
              tunnel: [w209 w212] -> w208
              tunnel: w206 -> [w209 w211]
              tunnel: w204 -> [_ w210]
              frame False {
              }
              frame True {
                n74 = invoke class="VI" method="FP.Close"(reference=w210, error in=w211) -> (error out=w212:errorcluster)  [unwired: 1 in, 2 out]
              }
            }
          }
          frame "Hidden", "Hide" {
            w213 = T3."Hidden" ("State")
            n75 = property class="VI"(reference=w219, error in=w218) -> (reference out=w216:refnum<vi>, error out=w217:errorcluster, "FP.State"=w215:T3)
            n76 = Not Equal?(x=w215, y=w213) -> (x != y?=w214:bool)
            n77 = case shown="True" w214 {
              tunnel: [w224 w225] -> w220
              tunnel: w217 -> [w223 w225]
              tunnel: w216 -> [w222 _]
              tunnel: w213 -> [w221 _]
              frame True {
                n78 = invoke class="VI" method="FP.Open"(reference=w222, error in=w223, "State"=w221) -> (error out=w224:errorcluster)  [unwired: 2 in, 4 out]
              }
              frame False {
              }
            }
          }
          frame "Minimize", "Minimized" {
            w226 = T3."Minimized" ("State")
            n79 = property class="VI"(reference=w232, error in=w231) -> (reference out=w229:refnum<vi>, error out=w230:errorcluster, "FP.State"=w228:T3)
            n80 = Not Equal?(x=w228, y=w226) -> (x != y?=w227:bool)
            n81 = case shown="True" w227 {
              tunnel: [w237 w238] -> w233
              tunnel: w230 -> [w236 w238]
              tunnel: w229 -> [w235 _]
              tunnel: w226 -> [w234 _]
              frame True {
                n82 = invoke class="VI" method="FP.Open"(reference=w235, error in=w236, "State"=w234) -> (error out=w237:errorcluster)  [unwired: 2 in, 4 out]
              }
              frame False {
              }
            }
          }
          frame "Maximize", "Maximized" {
            w239 = T3."Maximized" ("State")
            n83 = property class="VI"(reference=w245, error in=w244) -> (reference out=w242:refnum<vi>, error out=w243:errorcluster, "FP.State"=w241:T3)
            n84 = Not Equal?(x=w241, y=w239) -> (x != y?=w240:bool)
            n85 = case shown="True" w240 {
              tunnel: [w250 w251] -> w246
              tunnel: w243 -> [w249 w251]
              tunnel: w242 -> [w248 _]
              tunnel: w239 -> [w247 _]
              frame True {
                n86 = invoke class="VI" method="FP.Open"(reference=w248, error in=w249, "State"=w247) -> (error out=w250:errorcluster)  [unwired: 2 in, 4 out]
              }
              frame False {
              }
            }
          }
        }
        n87 = call <vilib>:"Add State(s) to Queue__jki_lib_state_machine.vi"("State(s) in (\"\")"=w186) -> ("States Out"=w185:string)  [unwired: 14 in]
      }
      frame "---------- Macro ----------" {
        # "Do not put any code in this frame.\n(It is a separator no-op. You can make a copy of this frame to create a new Macro frame)"
        n88 = call <vilib>:"Add State(s) to Queue__jki_lib_state_machine.vi"("State(s) in (\"\")"=w255) -> ("States Out"=w254:string)  [unwired: 14 in]
      }
      frame "Macro: Initialize" {
        w256 = "Data: Initialize\nInitialize Core Data\nUI: Initialize\nUI: EnDis Load>>Disable\nUI: Front Panel State >> Open\nAdams 6224: Init"  # Data: Initialize Initialize Core Data UI: Initialize UI: EnDis Load>>Disable UI: Front Panel State >> Open Adams 6224: Init
        # "Initialization Macro\n(This is called once, when the VI starts)"
        n89 = call <vilib>:"Add State(s) to Queue__jki_lib_state_machine.vi"("State(s) in Front (\"\")"=w256, "State(s) in (\"\")"=w260) -> ("States Out"=w259:string)  [unwired: 13 in]
      }
      frame "Macro: Measure Sensors" {
        # "Sequence for measuring sensors, converting to correct values and logging results (if required)."
        n90 = call <vilib>:"Add State(s) to Queue__jki_lib_state_machine.vi"("State(s) in Front (\"\")"="Adams 6017: Read AI\nPressure: Calculate Pressures\nTemperature: Calculate Temps\nLog: Write Data", "State(s) in (\"\")"=w265) -> ("States Out"=w264:string)  [unwired: 13 in]
      }
      frame "Macro: Exit" {
        # "Exit Macro\n(This is called once, when the VI exits)"
        n91 = Unbundle By Name(w272) -> ("Core.Close Panel on Exit?"=w267:bool)
        n92 = call <vilib>:"Conditional State String__jki_lib_state_machine.vi"("Do State(s)?"=w267, "State"="UI: Front Panel State >> Close") -> ("State Out"=w266:string)  [unwired: 7 in]
        n93 = call <vilib>:"Add State(s) to Queue__jki_lib_state_machine.vi"("State(s) in (\"\")"=w266, "State(s) at Back (\"\")"="Adams 6224: Close\nUI: Uninitialize\nData: Cleanup\nExit") -> ("States Out"=w270:string)  [unwired: 13 in]
        n94 = call <vilib>:"Add State(s) to Queue__jki_lib_state_machine.vi"("State(s) in Front (\"\")"=w270, "State(s) in (\"\")"=w274) -> ("States Out"=w273:string)  [unwired: 13 in]
      }
      frame "---------- Adams 6017 ----------" {
        # "Template Separator\n(You can make a copy of, or modify, this frame)"
        n95 = call <vilib>:"Add State(s) to Queue__jki_lib_state_machine.vi"("State(s) in (\"\")"=w278) -> ("States Out"=w277:string)  [unwired: 14 in]
      }
      frame "Adams 6017: Init" {
        # "#6017 IP address"
        # "Initialise the modbus connection to the Adams 6017 module"
        n96 = call "Adams Connect.vi"("Module Address"="IP address of 6017", "error in (no error)"=w284) -> ("Module Ref"=w279:refnum<class "Modbus Master.lvclass">, "error out"=w283:errorcluster)  [unwired: 12 in]
        n97 = Bundle By Name(cluster=w281, "6017 Ref"=w279) -> (w280:T9)
        n98 = call <vilib>:"Add State(s) to Queue__jki_lib_state_machine.vi"("State(s) in (\"\")"=w286) -> ("States Out"=w285:string)  [unwired: 14 in]
      }
      frame "Adams 6017: Read AI" {
        # "Read back AI register and convert to correct voltage/current values. Record a timestamp for logging purposes."
        n99 = Unbundle By Name(w295) -> ("Channel Ranges"=w288:T8[], "6017 Ref"=w296:refnum<class "Modbus Master.lvclass">, "Simulate Data"=w287:bool)
        n100 = case shown="False" w287 {
          tunnel: w297 -> [w307 w357]
          tunnel: w296 -> [w306 w358]
          tunnel: [w305 w358] -> w293
          tunnel: w288 -> [w303 _]
          tunnel: [w301 w356] -> w292
          tunnel: [w300 w354] -> w291
          frame False {
            n101 = call "Get AI.vi"("Module Ref"=w306, "error in (no error)"=w307) -> ("Modbus master out"=w305:refnum<class "Modbus Master.lvclass">, "AI Measurment"=w302:u16[], "error out"=w304:errorcluster)  [unwired: 11 in]
            n102 = for {
              tunnel: w304 -> [w310]
              tunnel: w303 -> [w312] mode=indexing
              tunnel: w302 -> [w311] mode=indexing
              tunnel: [w309] -> w301
              tunnel: [w308] -> w300 mode=indexing
              # "Use the range register value to convert the \nAI register value to the correct voltage/current"
              n103 = case shown="386" w312 {
                tunnel: w311 -> [_ w317 w320 w323 w326 w329 w332 w335 w338 w341 w344 w347 w350 w352]
                tunnel: w310 -> [w314 w315 w318 w321 w324 w327 w330 w333 w336 w339 w342 w345 w348 w353]
                tunnel: [w314 w315 w318 w321 w324 w327 w330 w333 w336 w339 w342 w345 w348 w353] -> w309
                tunnel: [0.0 ("Current mA") w316 w319 w322 w325 w328 w331 w334 w337 w340 w343 w346 w349 w351] -> w308
                frame 0, Default {
                }
                frame 259 {
                  n104 = call "+-150mV Conv.vi"("Register Value"=w317) -> ("Voltage mV"=w316:dbl)
                }
                frame 260 {
                  n105 = call "+-500mV Conv.vi"("Register Value"=w320) -> ("Voltage mV"=w319:dbl)
                }
                frame 261 {
                  n106 = call "0~150mV Conv.vi"("Register Value"=w323) -> ("Voltage mV"=w322:dbl)
                }
                frame 262 {
                  n107 = call "0~500mV Conv.vi"("Register Value"=w326) -> ("Voltage mV"=w325:dbl)
                }
                frame 320 {
                  n108 = call "+-1V Conv.vi"("Register Value"=w329) -> ("Voltage V"=w328:dbl)
                }
                frame 322 {
                  n109 = call "+-5V Conv.vi"("Register Value"=w332) -> ("Voltage V"=w331:dbl)
                }
                frame 323 {
                  n110 = call "+-10V Conv.vi"("Register Value"=w335) -> ("Voltage V"=w334:dbl)
                }
                frame 325 {
                  n111 = call "0~1V Conv.vi"("Register Value"=w338) -> ("Voltage V"=w337:dbl)
                }
                frame 327 {
                  n112 = call "0~5V Conv.vi"("Register Value"=w341) -> ("Voltage V"=w340:dbl)
                }
                frame 328 {
                  n113 = call "0~10V Conv.vi"("Register Value"=w344) -> ("Voltage V"=w343:dbl)
                }
                frame 385 {
                  n114 = call "+-20mA Conv.vi"("Register Value"=w347) -> ("Current mA"=w346:dbl)
                }
                frame 384 {
                  n115 = call "4~20mA Conv.vi"("Register Value"=w350) -> ("Current mA"=w349:dbl)
                }
                frame 386 {
                  n116 = call "0~20mA Conv.vi"("Register Value"=w352) -> ("Current mA"=w351:dbl)
                }
              }
            }
          }
          frame True {
            n117 = for {
              tunnel: w357 -> [w364]
              tunnel: [w364] -> w356
              tunnel: [w359] -> w354 mode=indexing
              tunnel: dbl[] [8.0, 7.0, 15.0, 6.0, 13.0, 12.0, 11.0, 0.5] -> [w361] mode=indexing
              n118 = call-poly <vilib>:"Random Number (Range).vi"("lower bound (0)"=0.0 ("upper bound (100)"), "upper bound (100)"=0.5) -> ("number"=w360:dbl)  [unwired: 9 in]
              n119 = Add(x=w361, y=w360) -> (x+y=w359:dbl)
            }
          }
        }
        n120 = Get Date/Time In Seconds() -> (seconds since 1Jan1904=w290:timestamp)
        n121 = To Double Precision Float(number=w290) -> (double precision float=w289:dbl)
        n122 = Bundle By Name(cluster=w295, "6017 Ref"=w293, "AI Measurment"=w291, "Timestamp"=w289) -> (w294:T9)
        n123 = call <vilib>:"Add State(s) to Queue__jki_lib_state_machine.vi"("State(s) in (\"\")"=w299) -> ("States Out"=w298:string)  [unwired: 14 in]
      }
      frame "Adams 6017: Set Ranges" {
        w365 = T8[] [328, 328, 384, 328, 384, 384, 384, 328] items=["+-150mV"=259, "+-500mV"=260, "0~150mV"=261, "0~500mV"=262, "+-1V"=320, "+-5V"=322, "+-10V"=323, "0~1V"=325, "0~5V"=327, "0~10V"=328, "+-20mA"=385, "4~20mA"=384, "0~20mA"=386]  # Channel Ranges
        # "Set the AI channel ranges"
        n124 = Unbundle By Name(w368) -> ("6017 Ref"=w370:refnum<class "Modbus Master.lvclass">)
        n125 = call "Set AI Ranges.vi"("Module Ref"=w370, "Channel Ranges"=w365, "error in (no error)"=w371) -> ("Modbus master out"=w366:refnum<class "Modbus Master.lvclass">, "error out"=w369:errorcluster)  [unwired: 11 in]
        n126 = Bundle By Name(cluster=w368, "6017 Ref"=w366, "Channel Ranges"=w365) -> (w367:T9)
        n127 = call <vilib>:"Add State(s) to Queue__jki_lib_state_machine.vi"("State(s) in (\"\")"=w373) -> ("States Out"=w372:string)  [unwired: 14 in]
      }
      frame "Adams 6017: Set DO" {
        # "Enable/disable the hydrolic load"
        n128 = Unbundle By Name(w379) -> ("6017 Ref"=w381:refnum<class "Modbus Master.lvclass">)
        n129 = case shown="\"Enable\"" w376 {
          tunnel: [FALSE TRUE] -> w375
          tunnel: [FALSE FALSE] -> w374
          frame "Disable", Default {
          }
          frame "Enable" {
          }
        }
        n130 = call "Set DO.vi"("Module Ref"=w381, "Channel 0"=w375, "Channel 1"=w374, "error in (no error)"=w380) -> ("Modbus master out"=w378:refnum<class "Modbus Master.lvclass">, "error out"=w382:errorcluster)  [unwired: 10 in]
        n131 = Bundle By Name(cluster=w379, "6017 Ref"=w378) -> (w377:T9)
        n132 = call <vilib>:"Add State(s) to Queue__jki_lib_state_machine.vi"("State(s) in (\"\")"=w384) -> ("States Out"=w383:string)  [unwired: 14 in]
      }
      frame "Adams 6017: Close" {
        # "Close the modbus reference to the Adams 6017 module."
        n133 = Unbundle By Name(w391) -> ("6017 Ref"=w392:refnum<class "Modbus Master.lvclass">)
        n134 = call "Adams Close.vi"("Modbus master in"=w392, "error in (no error)"=w394) -> ("error out"=w393:errorcluster)  [unwired: 13 in]
        n135 = Bundle By Name(cluster=w391, "6017 Ref"=refnum<class "Modbus Master.lvclass"> refnum) -> (w390:T9)
        n136 = call <vilib>:"Add State(s) to Queue__jki_lib_state_machine.vi"("State(s) in (\"\")"=w396) -> ("States Out"=w395:string)  [unwired: 14 in]
      }
      frame "---------- Adams 6224 ----------" {
        # "Template Separator\n(You can make a copy of, or modify, this frame)"
        n137 = call <vilib>:"Add State(s) to Queue__jki_lib_state_machine.vi"("State(s) in (\"\")"=w400) -> ("States Out"=w399:string)  [unwired: 14 in]
      }
      frame "Adams 6224: Init" {
        # "#6224 IP address"
        # "Initialise the modbus connection to the Adams 6224 module"
        n138 = call "Adams Connect.vi"("Module Address"="192.168.201.10", "error in (no error)"=w405) -> ("Module Ref"=w401:refnum<class "Modbus Master.lvclass">, "error out"=w404:errorcluster)  [unwired: 12 in]
        n139 = Bundle By Name(cluster=w403, "6224 Ref"=w401) -> (w402:T9)
        n140 = call <vilib>:"Add State(s) to Queue__jki_lib_state_machine.vi"("State(s) in (\"\")"=w408) -> ("States Out"=w407:string)  [unwired: 14 in]
      }
      frame "Adams 6224: Set AO" {
        w409 = T11 148 items=["+-5V"=142, "+-10V"=143, "0~5V"=147, "0~10V"=148] ("Voltage Output range")
        # "Convert from % to 10V range"
        # "Set the analogue out voltage to control the proportional load valve. Range is 0-10 volts."
        n141 = Unbundle By Name(w421) -> ("6224 Ref"=w418:refnum<class "Modbus Master.lvclass">, "Load Percentage"=w416:u32)
        n142 = To Double Precision Float(number=w416) -> (double precision float=w410:dbl)
        n143 = Divide(x=w410, y=100.0) -> (x/y=w414:dbl)
        n144 = Multiply(x=w414, y=10.0) -> (x*y=w412:dbl)
        n145 = call "Set AO.vi"("Module Ref"=w418, "Analogue Voltage Out"=w412, "Voltage Output range"=w409, "Channel"=enum16{"AO0.V+", "AO1.V+", "AO2.V+", "AO3.V+"}."AO0.V+", "error in (no error)"=w419) -> ("Modbus master out"=w417:refnum<class "Modbus Master.lvclass">, "error out"=w420:errorcluster)  [unwired: 9 in]
        n146 = Bundle By Name(cluster=w421, "6224 Ref"=w417) -> (w422:T9)
        n147 = call <vilib>:"Add State(s) to Queue__jki_lib_state_machine.vi"("State(s) in (\"\")"=w424) -> ("States Out"=w423:string)  [unwired: 14 in]
      }
      frame "Adams 6224: Close" {
        # "Close the modbus reference to the Adams 6224 module."
        n148 = Unbundle By Name(w426) -> ("6224 Ref"=w428:refnum<class "Modbus Master.lvclass">)
        n149 = call "Adams Close.vi"("Modbus master in"=w428, "error in (no error)"=w430) -> ("error out"=w429:errorcluster)  [unwired: 13 in]
        n150 = Bundle By Name(cluster=w426, "6224 Ref"=refnum<class "Modbus Master.lvclass"> refnum ("6017 Ref")) -> (w425:T9)
        n151 = call <vilib>:"Add State(s) to Queue__jki_lib_state_machine.vi"("State(s) in (\"\")"=w432) -> ("States Out"=w431:string)  [unwired: 14 in]
      }
      frame "---------- Pressure ----------" {
        # "Template Separator\n(You can make a copy of, or modify, this frame)"
        n152 = call <vilib>:"Add State(s) to Queue__jki_lib_state_machine.vi"("State(s) in (\"\")"=w436) -> ("States Out"=w435:string)  [unwired: 14 in]
      }
      frame "Pressure: Calculate Pressures" {
        # "Channels 1-4"
        # "Convert the analogue in voltage/currents to the appropriate pressure value. Add the converted values to the log data array."
        n153 = Unbundle By Name(w441) -> ("Log Data"=w437:dbl[], "Timestamp"=w438:dbl, "AI Measurment"=w452:dbl[])
        n154 = Index Array(array=w452, index #1=0 ("index")) -> (element #1=w450:dbl, element #2=w449:dbl, element #3=w447:dbl, element #4=w448:dbl)  [unwired: 3 in]
        n155 = call "0~10v 250bar.vi"("Voltage V"=w448) -> ("Pressure bar"=w442:dbl)
        "Load Pressure" <- w442
        n156 = call "0~10v 250bar.vi"("Voltage V"=w450) -> ("Pressure bar"=w445:dbl)
        "Prefilter Pressure" <- w445
        n157 = call "0~10v 250bar.vi"("Voltage V"=w449) -> ("Pressure bar"=w444:dbl)
        "Post Filter Pressure" <- w444
        n158 = call "4~20mA 10bar.vi"("Current mA"=w447) -> ("Pressure bar"=w443:dbl)
        "Cardev Pressure" <- w443
        n159 = Build Array (concatenate)(w437, w438, w445, w444, w443, w442) -> (w439:dbl[])
        n160 = Bundle("Pressure bar"=w445, "Pressure bar"=w444, "Pressure bar"=w443, "Pressure bar"=w442) -> (→"Pressures":T2)  [unwired: 1 in]
        n161 = Bundle By Name(cluster=w441, "Log Data"=w439) -> (w440:T9)
        n162 = call <vilib>:"Add State(s) to Queue__jki_lib_state_machine.vi"("State(s) in (\"\")"=w455) -> ("States Out"=w454:string)  [unwired: 14 in]
      }
      frame "---------- Temperature ----------" {
        # "Template Separator\n(You can make a copy of, or modify, this frame)"
        n163 = call <vilib>:"Add State(s) to Queue__jki_lib_state_machine.vi"("State(s) in (\"\")"=w459) -> ("States Out"=w458:string)  [unwired: 14 in]
      }
      frame "Temperature: Calculate Temps" {
        # "Channel 5, 6 and 8"
        # "Convert the analogue in voltage/currents to the appropriate temperature value. Add the converted values to the log data array."
        n164 = Unbundle By Name(w462) -> ("AI Measurment"=w473:dbl[])
        n165 = Unbundle By Name(w462) -> ("Log Data"=w466:dbl[])
        n166 = Index Array(array=w473, index #1=4 ("index"), index #3=7 ("index")) -> (element #1=w470:dbl, element #2=w469:dbl, element #3=w468:dbl)  [unwired: 1 in]
        n167 = call "4~20mA 100C.vi"("Current mA"=w469) -> ("Temperature °C"=w464:dbl)
        "Post Cooler Temp" <- w464
        n168 = call "4~20mA 100C.vi"("Current mA"=w470) -> ("Temperature °C"=w465:dbl)
        "Load Manifold Temp" <- w465
        n169 = call "NTC Thermistor lookup.vi"("Voltage Out"=w468) -> ("Temperature °C"=w463:dbl)
        "Motor Temp" <- w463
        n170 = Bundle("Temperature °C"=w465, "Temperature °C"=w464, "Temperature °C"=w463) -> (→"Temperatures":T12)  [unwired: 1 in]
        n171 = Build Array (concatenate)(w466, w465, w464, w463) -> (w460:dbl[])
        n172 = Bundle By Name(cluster=w462, "Log Data"=w460) -> (w461:T9)
        n173 = call <vilib>:"Add State(s) to Queue__jki_lib_state_machine.vi"("State(s) in (\"\")"=w476) -> ("States Out"=w475:string)  [unwired: 14 in]
      }
      frame "---------- ICM ----------" {
        n174 = call <vilib>:"Add State(s) to Queue__jki_lib_state_machine.vi"("State(s) in (\"\")"=w480) -> ("States Out"=w479:string)  [unwired: 14 in]
      }
      frame "ICM: Connect" {
        # "Initialise the serial modbus connection to the ICM 4.0 module"
        n175 = call "ICM Connect.vi"("Com Port"=refnum<visa-resource-name> refnum, "error in (no error)"=w486) -> ("ICM Ref"=w481:refnum<class "Modbus Master.lvclass">, "error out"=w484:errorcluster)  [unwired: 12 in]
        n176 = Bundle By Name(cluster=w483, "ICM Ref"=w481) -> (w482:T9)
        n177 = call <vilib>:"Add State(s) to Queue__jki_lib_state_machine.vi"("State(s) in (\"\")"=w488) -> ("States Out"=w487:string)  [unwired: 14 in]
      }
      frame "ICM: Close" {
        # "Close the serial modbus reference to the ICM 4.0 module."
        n178 = Unbundle By Name(w493) -> ("ICM Ref"=w490:refnum<class "Modbus Master.lvclass">)
        n179 = call "ICM Close.vi"("ICM Ref"=w490, "error in (no error)"=w491) -> ("error out"=w492:errorcluster)  [unwired: 13 in]
        n180 = Bundle By Name(cluster=w493, "ICM Ref"=refnum<class "Modbus Master.lvclass"> refnum) -> (w494:T9)
        n181 = call <vilib>:"Add State(s) to Queue__jki_lib_state_machine.vi"("State(s) in (\"\")"=w496) -> ("States Out"=w495:string)  [unwired: 14 in]
      }
      frame "ICM: ICM Results" {
        # "Read back the ISO 4066 results values from the ICM 4.0 module. Add the results to the results log array."
        n182 = Unbundle By Name(w506) -> ("ICM Ref"=w503:refnum<class "Modbus Master.lvclass">, "Log Data"=w501:dbl[])
        n183 = call "Get Results Codes.vi"("ICM Ref In"=w503, "error in (no error)"=w504) -> ("ICM Ref Out"=w502:refnum<class "Modbus Master.lvclass">, ">=4 µ"=w499:dbl, ">=6 µ"=w498:dbl, ">=14 µ"=w497:dbl, "error out"=w505:errorcluster)  [unwired: 9 in]
        ">4µ" <- w499
        ">6µ" <- w498
        ">14µ" <- w497
        n184 = Build Array (concatenate)(w501, w499, w498, w497) -> (w500:dbl[])
        n185 = Bundle By Name(cluster=w506, "ICM Ref"=w502, "Log Data"=w500) -> (w507:T9)
        n186 = call <vilib>:"Add State(s) to Queue__jki_lib_state_machine.vi"("State(s) in (\"\")"=w509) -> ("States Out"=w508:string)  [unwired: 14 in]
      }
      frame "ICM: Get Test Time" {
        # "Read back the current test completion time from the ICM  4.0 module."
        n187 = Unbundle By Name(w515) -> ("ICM Ref"=w512:refnum<class "Modbus Master.lvclass">)
        n188 = call "Get Completion.vi"("ICM Ref In"=w512, "error in (no error)"=w513) -> ("ICM Ref Out"=w511:refnum<class "Modbus Master.lvclass">, "Completion %"=→"ICM Test":dbl, "error out"=w514:errorcluster)  [unwired: 11 in]
        n189 = Bundle By Name(cluster=w515, "ICM Ref"=w511) -> (w516:T9)
        n190 = call <vilib>:"Add State(s) to Queue__jki_lib_state_machine.vi"("State(s) in (\"\")"=w518) -> ("States Out"=w517:string)  [unwired: 14 in]
      }
      frame "ICM: Get Temperature" {
        # "Read back the current oil temperature form the ICM 4.0 module."
        n191 = Unbundle By Name(w524) -> ("ICM Ref"=w521:refnum<class "Modbus Master.lvclass">)
        n192 = call "Get Temperature.vi"("ICM Ref In"=w521, "error in (no error)"=w522) -> ("ICM Ref Out"=w520:refnum<class "Modbus Master.lvclass">, "Temperature °C"=→"Temperature":dbl, "error out"=w523:errorcluster)  [unwired: 11 in]
        n193 = Bundle By Name(cluster=w524, "ICM Ref"=w520) -> (w525:T9)
        n194 = call <vilib>:"Add State(s) to Queue__jki_lib_state_machine.vi"("State(s) in (\"\")"=w527) -> ("States Out"=w526:string)  [unwired: 14 in]
      }
      frame "---------- Log ----------" {
        n195 = call <vilib>:"Add State(s) to Queue__jki_lib_state_machine.vi"("State(s) in (\"\")"=w531) -> ("States Out"=w530:string)  [unwired: 14 in]
      }
      frame "Log: Write Data" {
        # "Write the current log data to the log file (.csv) if the write data flag has been set."
        n196 = Unbundle By Name(w535) -> ("Results File Path"=w538:path, "Log Data"=w537:dbl[], "Write Data"=w532:bool)
        n197 = case shown="True" w532 {
          tunnel: w539 -> [w542 w548]
          tunnel: w538 -> [_ w547]
          tunnel: w537 -> [_ w546]
          tunnel: [w542 w543] -> w536
          frame False {
          }
          frame True {
            n198 = call-poly <vilib>:"Write Delimited Spreadsheet.vi"("file path (dialog if empty)"=w547, "1D data"=w546, "append to file? (new file:F)"=TRUE, "error in (no error)"=w548, "delimiter (\\t)"="," ("delimiter (\\t)")) -> ("error out"=w543:errorcluster)  [unwired: 9 in, 1 out]
          }
        }
        n199 = Bundle By Name(cluster=w535, "Log Data"=dbl[] []) -> (w534:T9)
        n200 = call <vilib>:"Add State(s) to Queue__jki_lib_state_machine.vi"("State(s) in (\"\")"=w541) -> ("States Out"=w540:string)  [unwired: 14 in]
      }
      frame "Log: Build Log File Name" {
        # "Write header and create log file"
        # "Generate the log file name to include the current time date. Create the file and write a header to it."
        n201 = call <vilib>:"Space Constant.vi"() -> ("String"=w558:string)
        n202 = Format Date/Time String(time format string (%c)="%H%M%S-%d%m%y") -> (date/time string=w557:string)  [unwired: 2 in]
        n203 = Concatenate Strings("Log File Name", w558, w557, ".csv") -> (w560:string)
        n204 = Build Path(base path=path "C:/results/HPU Test", name or relative path=w560) -> (appended path=w553:path)
        n205 = call-poly <vilib>:"Write Delimited Spreadsheet.vi"("file path (dialog if empty)"=w553, "1D data"=string[] ["Timestamp", "Pre Filter Pressure", "Post Filter Pressure", "Cardev Pressure", "Load Pressure", "Load Temperature", "Cooler Temperature", "Motor Temperature", ">4µ", ">6µ", ">14µ"], "error in (no error)"=w552, "delimiter (\\t)"="," ("delimiter (\\t)")) -> ("error out"=w551:errorcluster)  [unwired: 10 in, 1 out]
        n206 = Bundle By Name(cluster=w555, "Results File Path"=w553) -> (w554:T9)
        n207 = call <vilib>:"Add State(s) to Queue__jki_lib_state_machine.vi"("State(s) in (\"\")"=w564) -> ("States Out"=w563:string)  [unwired: 14 in]
      }
      frame "---------- Flow Meter ----------" {
        n208 = call <vilib>:"Add State(s) to Queue__jki_lib_state_machine.vi"("State(s) in (\"\")"=w568) -> ("States Out"=w567:string)  [unwired: 14 in]
      }
      frame "Flow Meter: Calculate Flow" {
        # "Need to be added in when we know what the\nflow rate at 20mA is set to."
        # "Convert the analogue in currents to the appropriate flow value. Add the converted values to the log data array."
        n209 = call <vilib>:"Add State(s) to Queue__jki_lib_state_machine.vi"("State(s) in (\"\")"=w572) -> ("States Out"=w571:string)  [unwired: 14 in]
      }
    }
  }
